vi "IPS Set Target Current Sweep Rate.vi"(4 "Error In":errorcluster={"status"=FALSE, "code"=1073676294, "source"="VISA Read in Prologix USB GPIB Command.vi"}, 6 "Current Sweep Rate (A/min)":dbl, 7 "VISA resource name":refnum<visa-resource-name>="COM3") -> (0 "Error Out":errorcluster={"status"=FALSE, "code"=1073676294, "source"="VISA Read in Prologix_GPIB_Sample.vi"}, 1 "Response":string, 3 "VISA resource name 2":refnum<visa-resource-name>="GPIB1::25::INSTR")   [LabVIEW 2016, in "IPS-120.lvlib"]
uses:
  IPS-120.lvlib
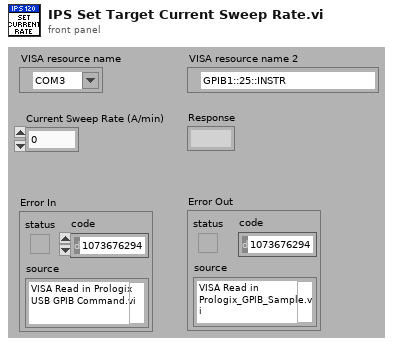
[diagram p1: front panel]
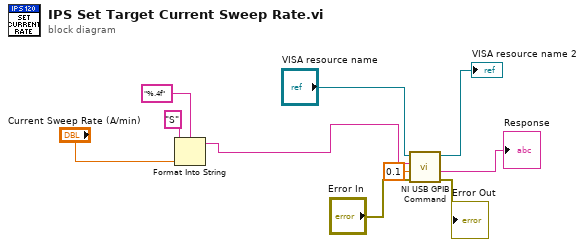
[diagram p0: block diagram]
diagram:
  n1 = Format Into String(format string="%.4f", initial string="S" ("string (\"\")"), "Current Sweep Rate (A/min)") -> (resulting string=w4:string)  [unwired: 1 in, 1 out]
  n2 = call "NI USB GPIB Command.vi"("Error In"="Error In", "Wait for instrument to respond (s)"=0.1, "String to Send"=w4, "VISA resource name"="VISA resource name") -> ("Error Out"=→"Error Out":errorcluster, "Return String from Device (Not all commands return a String)"=→"Response":string, "VISA resource name out"=→"VISA resource name 2":refnum<visa-resource-name>)  [unwired: 1 out]
